vi "Test_LEDs.vi"() -> ()   [LabVIEW 2014]
uses:
  <userlib>/UCSD Robotics Lab/Robotics-Cape/LV/libroboticscape.lvlib
panel:
  out "Timing Block":T1 {"Actual Hz" format="%#_3g"; "Dt" format="%#_4g"; "Average Hz" format="%#_4g"}
  in  "Green LED On/Off":bool
  in  "Red LED On/Off":bool
  out "Red LED":bool
  out "Green LED":bool
  out "Iteration counter":i32
  out "State":T2(ring)
  in  "stop":bool
  # "Always stop the VI using the rectangular STOP button above, never with the round stopsign (Abort)"
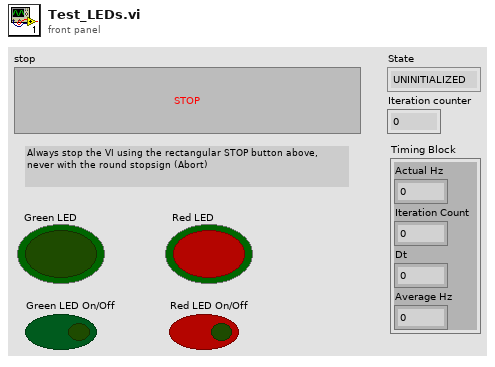
[diagram p1: front panel]
types:
  T1 = cluster{"Actual Hz":dbl, "Iteration Count":dbl, "Dt":dbl, "Average Hz":dbl}
  T2 = enum16{"UNINITIALIZED", "RUNNING", "PAUSED", "EXITING"}
  T3 = enum16{"UNINITIALIZED", "RUNING", "PAUSED", "EXITING"}
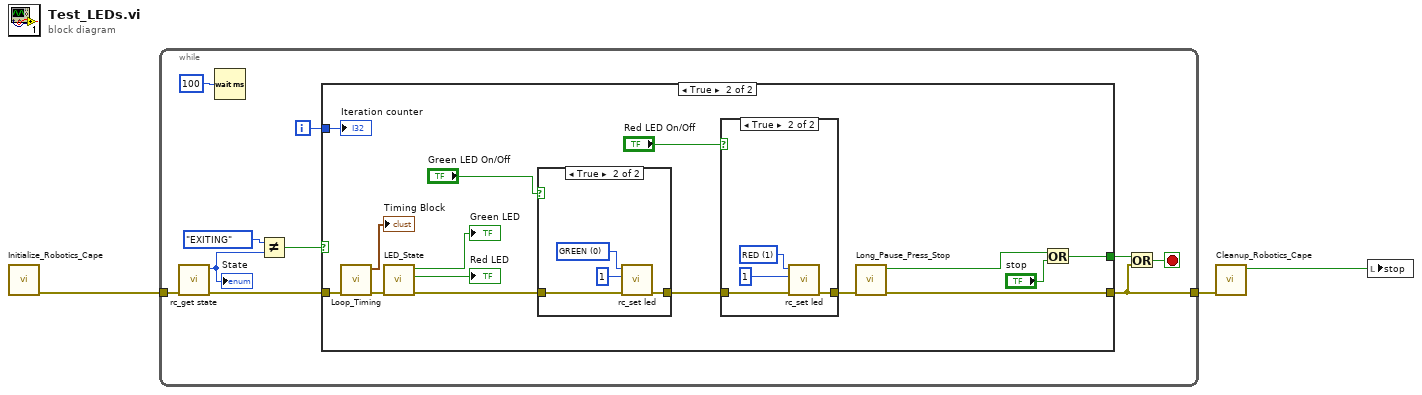
[diagram p0: block diagram]
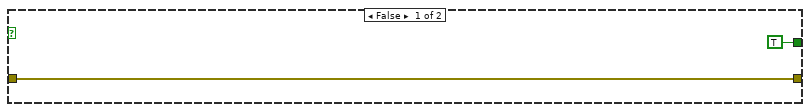
[diagram p2: hidden frame]
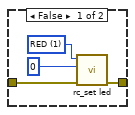
[diagram p3: hidden frame]
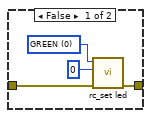
[diagram p4: hidden frame]
diagram:
  n1 = call "Initialize_Robotics_Cape.vi"() -> ("error out"=w3:errorcluster)  [unwired: 11 in]
  n2 = while {
    tunnel: w3 -> [w12]
    tunnel: [w5] -> w2
    i -> [w11]
    stop <- w13 stop-if-true
    n3 = call <userlib>:"rc_get state.vi"("error in (no error)"=w12) -> ("error out"=w10:errorcluster, "function return"=w8:u32)  [unwired: 9 in]
    "State" <- w8
    n4 = Wait (ms)(milliseconds to wait=u32 100) -> ()  [unwired: 1 out]
    n5 = Not Equal?(x=T3."EXITING" ("State 2"), y=w8) -> (x != y?=w9:bool)
    n6 = case shown="True" w9 {
      tunnel: w11 -> [_ w30]
      tunnel: w10 -> [w15 w23]
      tunnel: [w15 w19] -> w5
      tunnel: [TRUE ("stop") w16] -> w6
      frame False {
      }
      frame True {
        n7 = call "Loop_Timing.vi"("error in"=w23) -> ("error out"=w22:errorcluster, "Timing Block"=→"Timing Block":T1)  [unwired: 9 in]
        n8 = call "LED_State.vi"("error in (no error)"=w22) -> ("error out"=w27:errorcluster, "Red LED State"=→"Red LED":bool, "Green LED State"=→"Green LED":bool)  [unwired: 8 in]
        n9 = case shown="True" "Green LED On/Off" {
          tunnel: w27 -> [w40 w46]
          tunnel: [w39 w45] -> w26
          frame False {
            w42 = u32 0 items=["GREEN", "RED"] ("led")
            n10 = call <userlib>:"rc_set led.vi"("error in (no error)"=w40, "state"=0, "led"=w42) -> ("error out"=w39:errorcluster)  [unwired: 7 in, 1 out]
          }
          frame True {
            w43 = u32 0 items=["GREEN", "RED"] ("led")
            n11 = call <userlib>:"rc_set led.vi"("error in (no error)"=w46, "state"=1, "led"=w43) -> ("error out"=w45:errorcluster)  [unwired: 7 in, 1 out]
          }
        }
        n12 = case shown="True" "Red LED On/Off" {
          tunnel: w26 -> [w32 w38]
          tunnel: [w31 w37] -> w20
          frame False {
            w34 = u32 1 items=["GREEN", "RED"] ("led")
            n13 = call <userlib>:"rc_set led.vi"("error in (no error)"=w32, "state"=0, "led"=w34) -> ("error out"=w31:errorcluster)  [unwired: 7 in, 1 out]
          }
          frame True {
            w35 = u32 1 items=["GREEN", "RED"] ("led")
            n14 = call <userlib>:"rc_set led.vi"("error in (no error)"=w38, "state"=1, "led"=w35) -> ("error out"=w37:errorcluster)  [unwired: 7 in, 1 out]
          }
        }
        n15 = call "Long_Pause_Press_Stop.vi"("error in (no error)"=w20) -> ("error out"=w19:errorcluster, "Stop"=w17:bool)  [unwired: 9 in]
        n16 = Or(x=w17, y="stop") -> (x .or. y?=w16:bool)
        "Iteration counter" <- w30
      }
    }
    n17 = Or(x=w6, y=w5) -> (x .or. y?=w13:bool)
  }
  n18 = call "Cleanup_Robotics_Cape.vi"("error in (no error)"=w2) -> ("Stop Local Variabl"=w1:bool)  [unwired: 9 in, 1 out]
  n19 = local write "stop"(w1) -> ()
